vi "array_unit_conversion.vi"(2 "inverse function (arb. unit to s)?":bool=TRUE, 3 "delay array 2":dbl[](array[numeric]), 4 "delay array":dbl[](array[numeric]), 5 "time unit":enum16{"s", "ms", "us", "ns"}(ring)) -> (0 "output 2":dbl[](array[numeric]), 1 "output":dbl[](array[numeric]))   [LabVIEW 2012]
doc: "This VI converts a delay array from seconds to the specified unit."
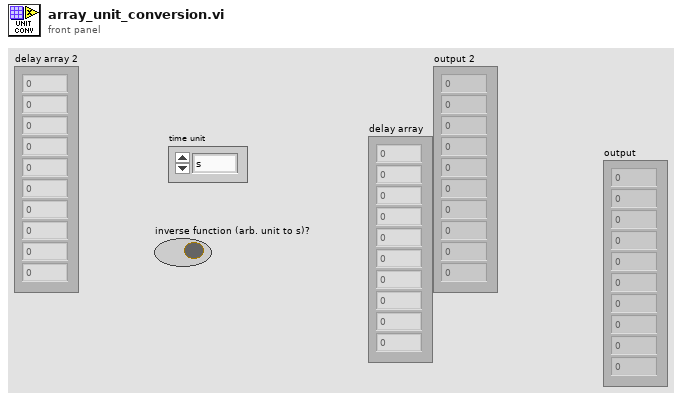
[diagram p1: front panel]
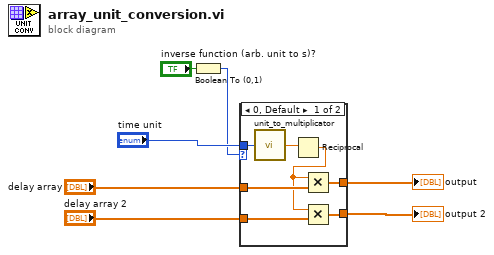
[diagram p0: block diagram]
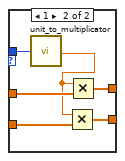
[diagram p2: hidden frame]
diagram:
  n1 = Boolean To (0,1)(Boolean="inverse function (arb. unit to s)?") -> (0, 1=w5:i16)
  n2 = case shown="0, Default" w5 {
    tunnel: "time unit" -> [w14 w20]
    tunnel: [w13 w19] -> w3
    tunnel: "delay array" -> [w12 w18]
    tunnel: "delay array 2" -> [w9 w17]
    tunnel: [w10 w15] -> w1
    frame 0, Default {
      n3 = call "unit_to_multiplicator.vi"("time unit"=w14) -> ("multiplicator"=w11:dbl)
      n4 = Reciprocal(x=w11) -> (1/x=w8:dbl)
      n5 = Multiply(x=w8, y=w12) -> (x*y=w13:dbl[])
      n6 = Multiply(x=w8, y=w9) -> (x*y=w10:dbl[])
    }
    frame 1 {
      n7 = call "unit_to_multiplicator.vi"("time unit"=w20) -> ("multiplicator"=w16:dbl)
      n8 = Multiply(x=w16, y=w17) -> (x*y=w15:dbl[])
      n9 = Multiply(x=w16, y=w18) -> (x*y=w19:dbl[])
    }
  }
  "output" <- w3
  "output 2" <- w1
